vi "GetCellStrColor.vi"(7 "Color":u32, 8 "error in (no error)":errorcluster, 10 "Hdr Name":T1, 11 "Tachometer in":refnum<class "Tachometer.lvclass">) -> (0 "error out":errorcluster, 1 "Cell String":string, 2 "Cell Color":u32, 3 "Tachometer out":refnum<class "Tachometer.lvclass">)   [LabVIEW 2018, in "Measurement Channels.lvlib" / "Tachometer.lvclass"]
uses:
  Tachometer.lvclass
  Common/Controls/HeaderNames.ctl
  Tachometer.lvclass/Tachometer.ctl
  Class Frequency/Frequency.lvclass
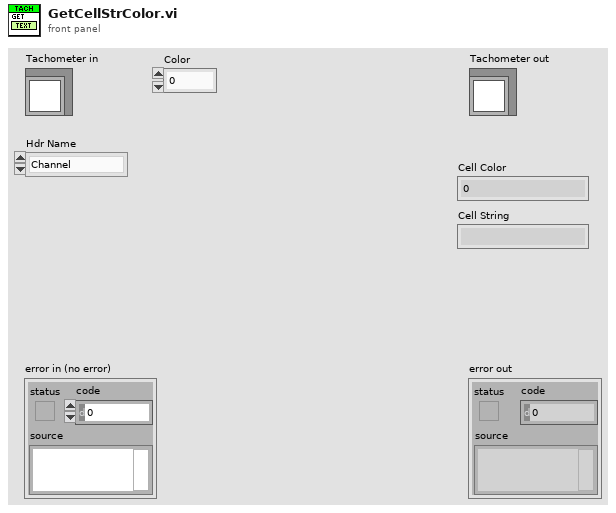
[diagram p1: front panel]
types:
  T1 = typedef "HeaderNames.ctl" = enum16{"Channel", "Device", "Spacer", "Description", "MB", "Range", "Terminal", "Coupling", "Thresh (V)", "Pulse/Rev", "Slope", "Min EU", "Min RPM", "mV/EU", "Iex", "Temp Units", "Type", "CJC Src", "CJC Val", "Ro", "Wire Cfg", "Strain Mode", "Vex", "Bridge Type", "GF", "Gauge Res", "Poisson", "Lead Res", "Init Strain", "GAF", "Scale", "Offset", "Unit (EU)", "dB?", "dB Ref", "Cal Mag", "Cal Units", "Max Temp", "Min Temp", "Max Strain", "Min Strain"}
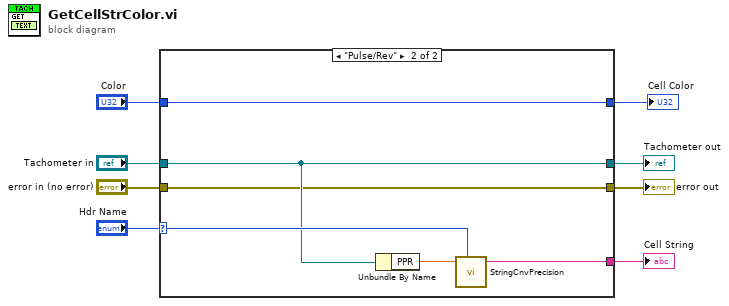
[diagram p0: block diagram]
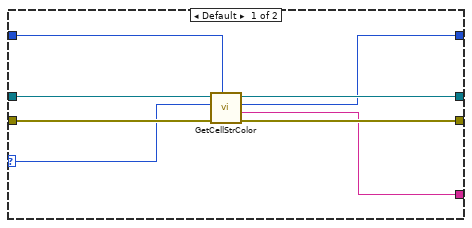
[diagram p2: hidden frame]
diagram:
  n1 = case shown="\"Pulse/Rev\"" "Hdr Name" {
    selector: "Hdr Name" -> [w10 w21]
    tunnel: [w12 w17] -> w3
    tunnel: "Color" -> [w9 w17]
    tunnel: "Tachometer in" -> [w16 w20]
    tunnel: "error in (no error)" -> [w15 w18]
    tunnel: [w14 w20] -> w5
    tunnel: [w13 w18] -> w4
    tunnel: [w11 w19] -> w2
    frame Default {
      n2 = call-parent "GetCellStrColor.vi"("Color"=w9, "error in (no error)"=w15, "Hdr Name"=w10, "Frequency in"=w16) -> ("error out"=w13:errorcluster, "Cell String"=w11:string, "Cell Color"=w12:u32, "Frequency out"=w14:refnum<class "Tachometer.lvclass">)  [unwired: 4 in]
    }
    frame "Pulse/Rev" {
      n3 = Unbundle By Name(w20) -> ("PPR"=w22:dbl)
      n4 = call "StringCnvPrecision.vi"("Number"=w22, "Header"=w21) -> ("Float String"=w19:string)  [unwired: 5 in]
    }
  }
  "error out" <- w4
  "Tachometer out" <- w5
  "Cell String" <- w2
  "Cell Color" <- w3
